vi "411x_Global.vi"() -> ()   [LabVIEW 2023, in "NI PXIe-411x PS Custom Device.lvlib"]
uses:
  NI PXIe-411x PS Custom Device.lvlib
panel:
  in  "411x Channel Page":string="10877fa4-c2d4-4222-826b-ae30f45b243a"
  in  "411x Page Disable GUID":string="afdabf9d-2f00-4ac4-aee0-3d42bf8ba41d"
  in  "Module":string="Module"
  in  "Initial C Value":string="Initial C Value"
  in  "Channel Name":string="Channel #"
  in  "411x Page GUID":string="c4962e37-b61c-419d-86ec-cab6a3f4360a"
  in  "Voltage Limit":string="Voltage Limit"
  in  "Current Limit":string="Current Limit"
  in  "Initial V Value":string="Initial V Value"
  in  "Sense":string="Sense"
  in  "IO Type":string="IO Type"
  in  "Channel #":string="Channel #"
  in  "Device Name":string="Device Name"
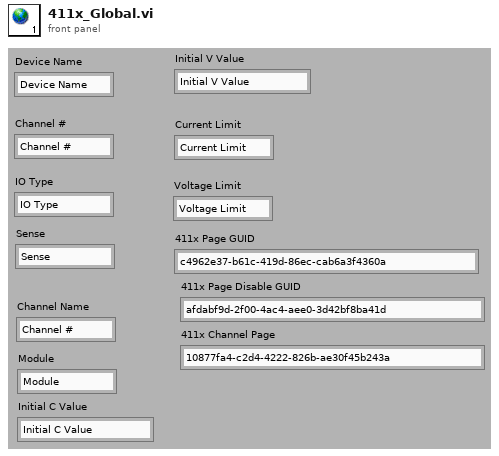
[diagram p1: front panel]
diagram:
